vi "SAVE PRODUCT IN DATABASE.vi"(8 "error in (no error)":errorcluster, 10 "PRODUCTS":T1) -> (0 "error out":errorcluster)   [LabVIEW 2019, in "CONFIGURATION.lvlib"]
doc: "HERE WE CAN UPDATE OUR DB OF PRODUCTS\n_____\nCreated using Delacor QMH Event Scripter 5.0.0.112."
uses:
  CONFIGURATION.lvlib
  DB_VENDING MACHINE/Type Defs/PRODUCTS.ctl
  SAVE PRODUCT IN DATABASE Argument--cluster.ctl
  DB_VENDING MACHINE/DB_VENDING MACHINE.lvlib
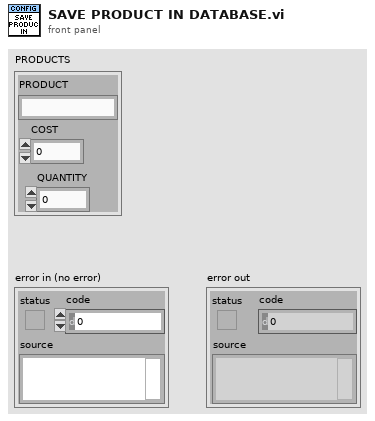
[diagram p1: front panel]
types:
  T1 = typedef "DB_VENDING MACHINE.lvlib/PRODUCTS.ctl" = cluster{"PRODUCT":string, "COST":dbl, "QUANTITY":i8}
  T2 = typedef "CONFIGURATION.lvlib/SAVE PRODUCT IN DATABASE Argument--cluster.ctl" = cluster{"PRODUCTS":T1}
  T3 = typedef "CONFIGURATION.lvlib/Request Events--cluster.ctl" = cluster{"Stop Module":refnum<user-event>, "Show Panel":refnum<user-event>, "Hide Panel":refnum<user-event>, "Get Module Execution Status":refnum<user-event>, "Show Diagram":refnum<user-event>, "SET CONFIGURATIO":refnum<user-event>, "UPDATE DB TO MONEY LIST":refnum<user-event>, "SAVE IN DB":refnum<user-event>, "SAVE PRODUCT IN DATABASE":refnum<user-event>, "UPDATE DB TO PRODUCT LIST":refnum<user-event>}
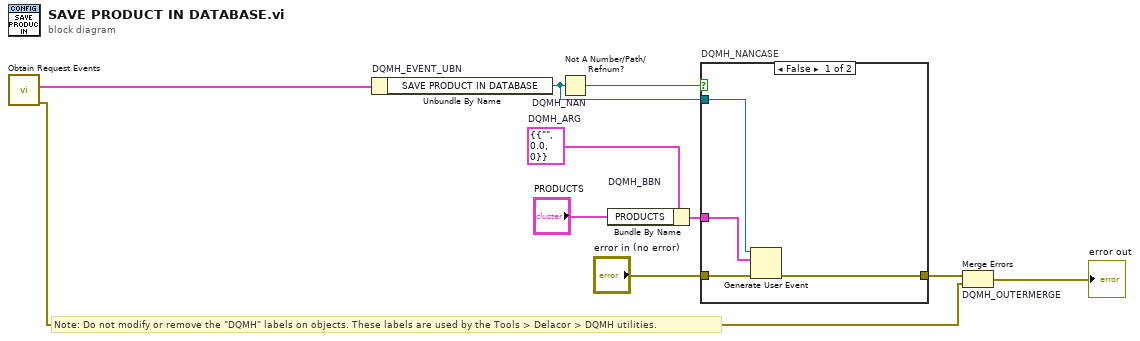
[diagram p0: block diagram]
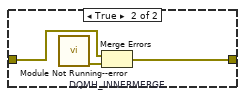
[diagram p2: hidden frame]
diagram:
  w4 = T2 {"PRODUCTS"={"PRODUCT"="", "COST"=0.0, "QUANTITY"=0}}  # DQMH_ARG
  # "Note: Do not modify or remove the \"DQMH\" labels on objects. These labels are used by the Tools > Delacor > DQMH utilities."
  n1 = call "Obtain Request Events.vi"() -> ("error out"=w2:errorcluster, "CONFIGURATION Request Events"=w1:T3)  [unwired: 10 in]
  n2 = Unbundle By Name "DQMH_EVENT_UBN"(w1) -> ("SAVE PRODUCT IN DATABASE"=w6:refnum<user-event>)
  n3 = Not A Number/Path/Refnum? "DQMH_NAN"(number/path/refnum=w6) -> (NaN/Path/Refnum?=w7:bool)
  n4 = Bundle By Name "DQMH_BBN"(cluster=w4, "PRODUCTS"="PRODUCTS") -> (w8:T2)
  n5 = case "DQMH_NANCASE" shown="False" w7 {
    tunnel: "error in (no error)" -> [w14 w17]
    tunnel: [w13 w16] -> w5
    tunnel: w6 -> [w12 _]
    tunnel: w8 -> [w11 _]
    frame False {
      n6 = Generate User Event(user event=w12, event data cluster=w11, error in=w14) -> (error out=w13:errorcluster)  [unwired: 1 in, 1 out]
    }
    frame True {
      n7 = call "Module Not Running--error.vi"() -> ("error out"=w15:errorcluster)  [unwired: 11 in]
      n8 = Merge Errors "DQMH_INNERMERGE"(w17, w15) -> (w16:errorcluster)
    }
  }
  n9 = Merge Errors "DQMH_OUTERMERGE"(w5, w2) -> (→"error out":errorcluster)
